vi "Query Trace Data.vi"(8 "error in (no error)":errorcluster, 11 "SA-ESA in":refnum<class "SA-ESA.lvclass">) -> (0 "error out":errorcluster, 1 "Level":dbl[](array[numeric]), 2 "Frequency/Time":dbl[](array[numeric]), 3 "SA-ESA out":refnum<class "SA-ESA.lvclass">)   [LabVIEW 2020, in "SA-ESA.lvclass"]
uses:
  SA-ESA.lvclass
  C:/Sandbox/RF Bench/Source Code/WiSpry Test Framework/Instruments/Instrument.lvclass
  C:/Sandbox/RF Bench/Source Code/WiSpry Test Framework/Instruments/Spectrum Analyzer/Spectrum Analyzer.lvclass
  Spectrum Analyzer.lvclass/Spectrum Analyzer.ctl
  Instrument.lvclass/Instrument.ctl
  Instrument.lvclass
  Spectrum Analyzer.lvclass
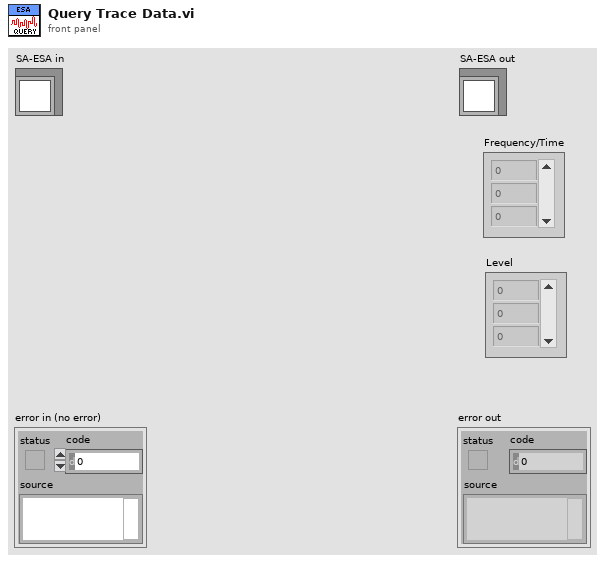
[diagram p1: front panel]
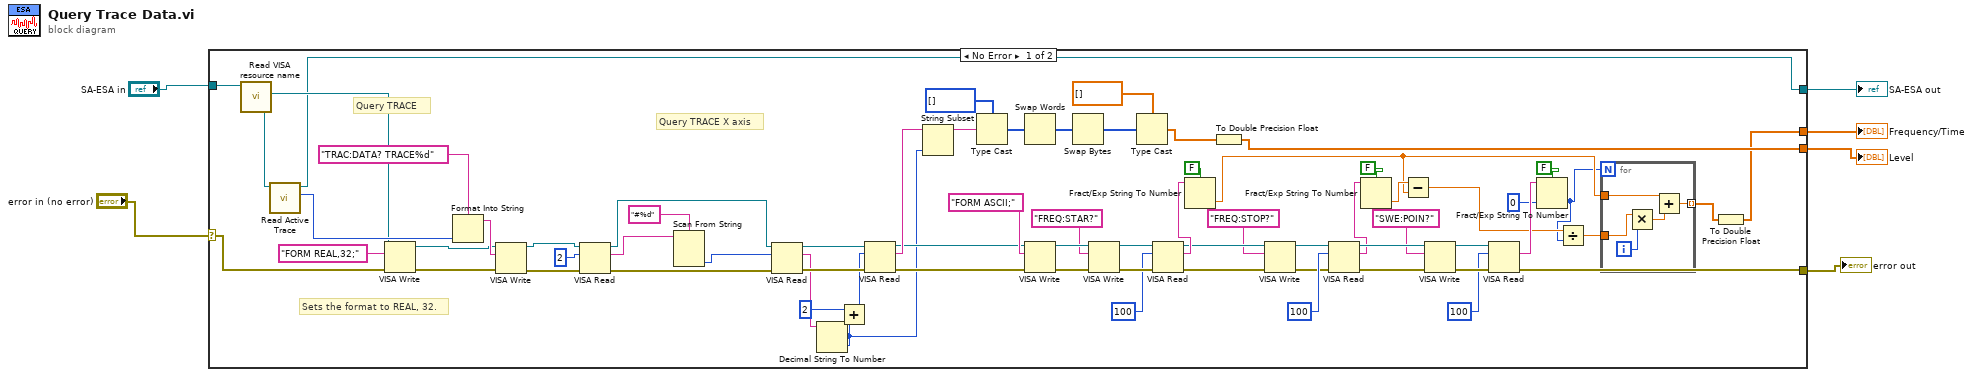
[diagram p0: block diagram]
diagram:
  n1 = case shown="No Error" "error in (no error)" {
    selector: "error in (no error)" -> [w48 w82]
    tunnel: "SA-ESA in" -> [w49 w83]
    tunnel: [w47 _] -> w4
    tunnel: [w46 _] -> w1
    tunnel: [w21 w82] -> w3
    tunnel: [w45 w83] -> w2
    frame No Error {
      # "Sets the format to REAL, 32."
      # "Query TRACE X axis"
      # "Query TRACE"
      n2 = call "Read VISA resource name.vi"("Instrument in"=w49) -> ("VISA resource name"=w62:refnum<visa-resource-name>, "Instrument out"=w76:refnum<class "SA-ESA.lvclass">)  [unwired: 9 in]
      n3 = call "Read Active Trace.vi"("Spectrum Analyzer in"=w76) -> ("Active Trace"=w66:u16, "Spectrum Analyzer out"=w45:refnum<class "SA-ESA.lvclass">)  [unwired: 9 in]
      n4 = VISA Write(VISA resource name=w62, write buffer="FORM REAL,32;", error in (no error)=w48) -> (VISA resource name out=w63:refnum<visa-resource-name>, error out=w64:errorcluster)  [unwired: 1 out]
      n5 = Format Into String(format string="TRAC:DATA? TRACE%d", w66) -> (resulting string=w74:string)  [unwired: 2 in, 1 out]
      n6 = VISA Write(VISA resource name=w63, write buffer=w74, error in (no error)=w64) -> (VISA resource name out=w72:refnum<visa-resource-name>, error out=w73:errorcluster)  [unwired: 1 out]
      n7 = VISA Read(VISA resource name=w72, byte count=u32 2, error in (no error)=w73) -> (VISA resource name out=w67:refnum<visa-resource-name>, read buffer=w71:string, error out=w69:errorcluster)  [unwired: 1 out]
      n8 = Scan From String(format string="#%d", input string=w71) -> (output 1=w60:i32)  [unwired: 3 in, 3 out]
      n9 = VISA Read(VISA resource name=w67, byte count=w60, error in (no error)=w69) -> (VISA resource name out=w58:refnum<visa-resource-name>, read buffer=w57:string, error out=w59:errorcluster)  [unwired: 1 out]
      n10 = Decimal String To Number(string=w57) -> (number=w7:i32)  [unwired: 2 in, 1 out]
      n11 = Add(x=2, y=w7) -> (x+y=w44:i32)
      n12 = VISA Read(VISA resource name=w58, byte count=w44, error in (no error)=w59) -> (VISA resource name out=w42:refnum<visa-resource-name>, read buffer=w56:string, error out=w41:errorcluster)  [unwired: 1 out]
      n13 = String Subset(string=w56, length (rest)=w7) -> (substring=w8:string)  [unwired: 1 in]
      n14 = Type Cast(type=i8[] [], x=w8) -> (*(type *) &x=w54:i8[])
      n15 = Swap Words(1:w54) -> (0:w53:i8[])
      n16 = VISA Write(VISA resource name=w42, write buffer="FORM ASCII;", error in (no error)=w41) -> (VISA resource name out=w39:refnum<visa-resource-name>, error out=w40:errorcluster)  [unwired: 1 out]
      n17 = Swap Bytes(anything=w53) -> (byte swapped=w52:i8[])
      n18 = VISA Write(VISA resource name=w39, write buffer="FREQ:STAR?", error in (no error)=w40) -> (VISA resource name out=w36:refnum<visa-resource-name>, error out=w37:errorcluster)  [unwired: 1 out]
      n19 = Type Cast(type=sgl[] [], x=w52) -> (*(type *) &x=w50:sgl[])
      n20 = VISA Read(VISA resource name=w36, byte count=u32 100, error in (no error)=w37) -> (VISA resource name out=w29:refnum<visa-resource-name>, read buffer=w34:string, error out=w27:errorcluster)  [unwired: 1 out]
      n21 = Fract/Exp String To Number(use system decimal point (T)=FALSE, string=w34) -> (number=w13:dbl)  [unwired: 2 in, 1 out]
      n22 = To Double Precision Float(number=w50) -> (double precision float=w47:dbl[])
      n23 = VISA Write(VISA resource name=w29, write buffer="FREQ:STOP?", error in (no error)=w27) -> (VISA resource name out=w31:refnum<visa-resource-name>, error out=w30:errorcluster)  [unwired: 1 out]
      n24 = VISA Read(VISA resource name=w31, byte count=u32 100, error in (no error)=w30) -> (VISA resource name out=w23:refnum<visa-resource-name>, read buffer=w16:string, error out=w22:errorcluster)  [unwired: 1 out]
      n25 = Fract/Exp String To Number(use system decimal point (T)=FALSE, string=w16) -> (number=w14:dbl)  [unwired: 2 in, 1 out]
      n26 = Subtract(x=w14, y=w13) -> (x-y=w12:dbl)
      n27 = VISA Write(VISA resource name=w23, write buffer="SWE:POIN?", error in (no error)=w22) -> (VISA resource name out=w25:refnum<visa-resource-name>, error out=w26:errorcluster)  [unwired: 1 out]
      n28 = VISA Read(VISA resource name=w25, byte count=u32 100, error in (no error)=w26) -> (read buffer=w19:string, error out=w21:errorcluster)  [unwired: 2 out]
      n29 = Fract/Exp String To Number(use system decimal point (T)=FALSE, string=w19, default (0 dbl)=0) -> (number=w11:i32)  [unwired: 1 in, 1 out]
      n30 = Divide(x=w12, y=w11) -> (x/y=w10:dbl)
      n31 = for {
        N: w11 -> [_]
        tunnel: w13 -> [w81]
        tunnel: w10 -> [w79]
        tunnel: [w77] -> w9 mode=indexing
        i -> [w80]
        n32 = Multiply(x=w79, y=w80) -> (x*y=w78:dbl)
        n33 = Add(x=w81, y=w78) -> (x+y=w77:dbl)
      }
      n34 = To Double Precision Float(number=w9) -> (double precision float=w46:dbl[])
    }
    frame Error {
    }
  }
  "error out" <- w3
  "SA-ESA out" <- w2
  "Level" <- w4
  "Frequency/Time" <- w1
